vi "Channel Count.vi"(8 "error in (no error)":errorcluster, 11 "Transfer Group Configuration in":T1={"name"="", "direction"=enum."Tx", "cycle timing"={"priority"=0, "decimation"=1, "offset"=0}, "Transfers"=[], "settings"=[]} {"Transfers"."channel configurations"."buffer offset" format="%d bytes"}) -> (0 "error out":errorcluster, 2 "total channel count":u64, 3 "Transfer Group Configuration out":T1={"name"="", "direction"=enum."Tx", "cycle timing"={"priority"=0, "decimation"=1, "offset"=0}, "Transfers"=[], "settings"=[]} {"Transfers"."channel configurations"."buffer offset" format="%d bytes"})   [LabVIEW 2017, in "DSF Core.lvlib"]
uses:
  DSF Core.lvlib
  Controls/DSF Engine Transfer Group Configuration.ctl
  Controls/DSF Direction.ctl
  Controls/DSF Timing Info.ctl
  Controls/DSF Engine Transfer Configuration.ctl
  Controls/DSF Byte Order.ctl
  Controls/DSF Engine Channel Configuration.ctl
  Controls/DSF Data Type.ctl
  Controls/DSF Settings Info.ctl
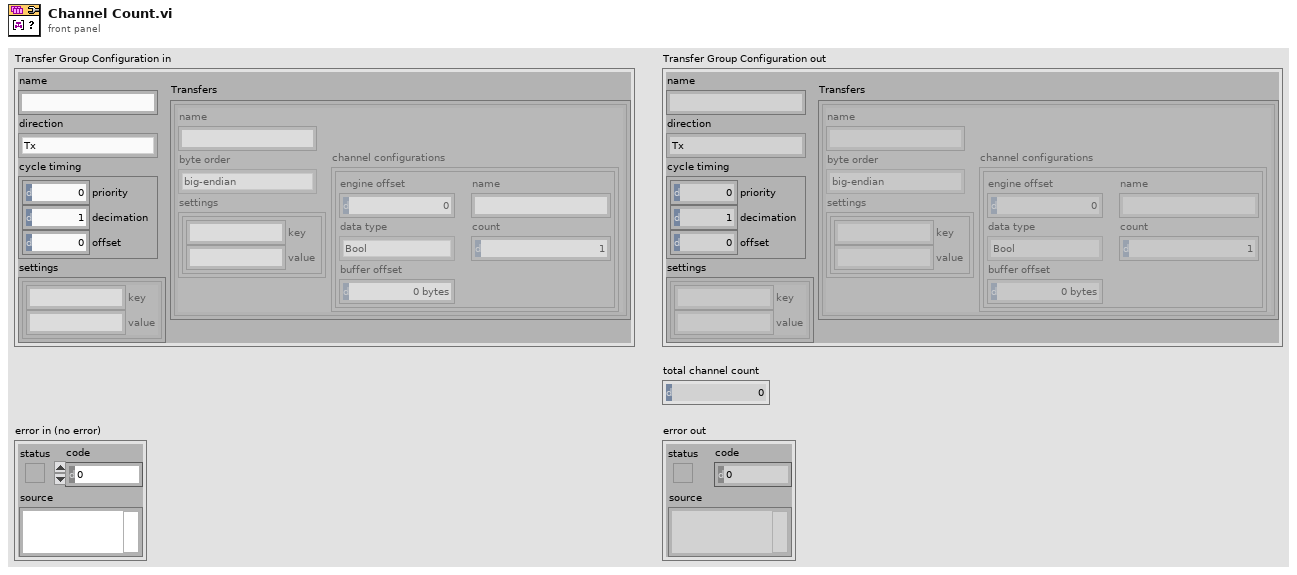
[diagram p1: front panel]
types:
  T1 = typedef "DSF Core.lvlib/DSF Engine Transfer Group Configuration.ctl" = cluster{"name":string, "direction":T2, "cycle timing":T3, "Transfers":T4[], "settings":T8}
  T2 = typedef "DSF Core.lvlib/DSF Direction.ctl" = enum8{"Tx", "Rx"}
  T3 = typedef "DSF Core.lvlib/DSF Timing Info.ctl" = cluster{"priority":u64, "decimation":u64, "offset":u64}
  T4 = typedef "DSF Core.lvlib/DSF Engine Transfer Configuration.ctl" = cluster{"name":string, "byte order":T5, "channel configurations":T6[], "settings":T8}
  T5 = typedef "DSF Core.lvlib/DSF Byte Order.ctl" = enum8{"big-endian", "little-endian"}
  T6 = typedef "DSF Core.lvlib/DSF Engine Channel Configuration.ctl" = cluster{"engine offset":u64, "name":string, "data type":T7, "count":u64, "buffer offset":u64}
  T7 = typedef "DSF Core.lvlib/DSF Data Type.ctl" = enum8{"Bool", "SGL", "DBL", "I8", "I16", "I32", "I64", "U8", "U16", "U32", "U64"}
  T8 = typedef "DSF Core.lvlib/DSF Settings Info.ctl" = cluster{"key":string, "value":string}[]
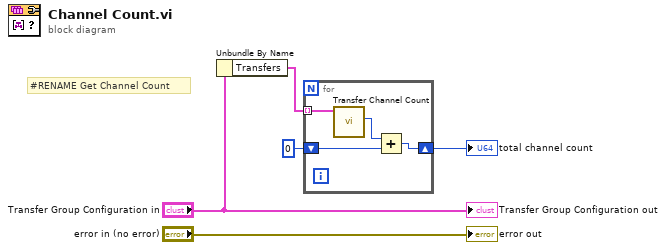
[diagram p0: block diagram]
diagram:
  # "#RENAME Get Channel Count"
  n1 = Unbundle By Name("Transfer Group Configuration in") -> ("Transfers"=w1:T4[])
  n2 = for {
    tunnel: w1 -> [w7] mode=indexing
    shift-right: [w9] -> w3
    shift-left: u64 0 -> [w8]
    n3 = call "Transfer Channel Count.vi"("Transfer Configuration in"=w7) -> ("total channel count"=w6:u64)  [unwired: 8 in, 2 out]
    n4 = Add(x=w6, y=w8) -> (x+y=w9:u64)
  }
  "total channel count" <- w3
  "error out" <- "error in (no error)"
  "Transfer Group Configuration out" <- "Transfer Group Configuration in"
